vi "CSTK_MCListbox_Designer.vi"(10 "应用程序:菜单启动:VI":string, 11 "应用程序引用（本地）":refnum<vi>) -> ()   [LabVIEW 2015, in "CSTK_MCListbox Designer.lvlib"]
uses:
  CSTK_MCListbox Designer.lvlib
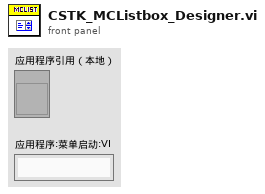
[diagram p1: front panel]
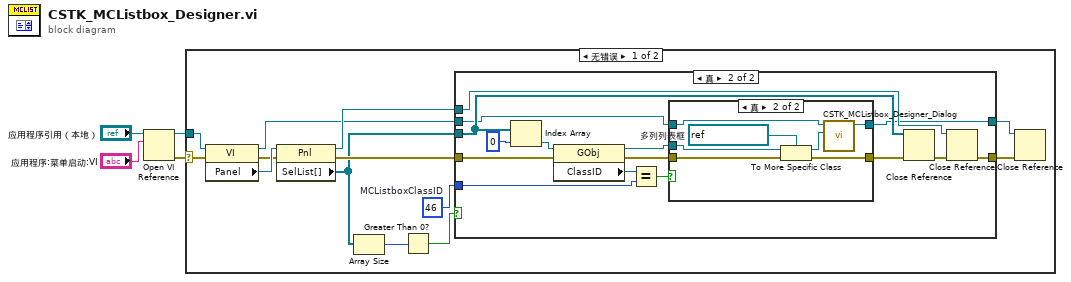
[diagram p0: block diagram]
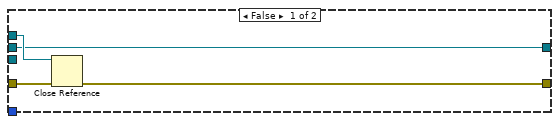
[diagram p2: hidden frame]
diagram:
  n1 = Open VI Reference(application reference (local)="应用程序引用（本地）", vi path="应用程序:菜单启动:VI") -> (vi reference=w1:refnum<vi>, error out=w2:errorcluster)  [unwired: 4 in]
  n2 = case shown="无错误" w2 {
    selector: w2 -> [w8 _]
    tunnel: w1 -> [w9 _]
    frame No Error {
      w10 = u32 46  # MCListboxClassID
      n3 = property class="VI"(reference=w9, error in=w8) -> (reference out=w6:refnum<vi>, error out=w16:errorcluster, "Panel"=w17:refnum<vi>)
      n4 = property class="Pnl"(reference=w17, error in=w16) -> (reference out=w12:refnum<vi>, error out=w13:errorcluster, "SelList[]"=w11:refnum<vi>[])
      n5 = Array Size(array=w11) -> (size(s)=w15:i32)
      n6 = Greater Than 0?(x=w15) -> (x > 0?=w14:bool)
      n7 = case shown="真" w14 {
        tunnel: w13 -> [w21 w34]
        tunnel: w12 -> [w20 w26]
        tunnel: w11 -> [_ w27]
        tunnel: w10 -> [_ w32]
        tunnel: [w19 w25] -> w7
        tunnel: w6 -> [w18 w23]
        tunnel: [w18 w22] -> w5
        frame False {
          n8 = Close Reference(reference=w20, error in (no error)=w21) -> (error out=w19:errorcluster)
        }
        frame True {
          n9 = Index Array(array=w27, index=0 ("索引")) -> (element=w35:refnum<vi>)
          n10 = property class="GObj"(reference=w35, error in=w34) -> (reference out=w24:refnum<vi>, error out=w30:errorcluster, "ClassID"=w33:u32)
          n11 = Equal?(x=w33, y=w32) -> (x = y?=w31:bool)
          n12 = case shown="真" w31 {
            tunnel: [w38 w41] -> w28
            tunnel: w30 -> [w38 w44]
            tunnel: w24 -> [_ w43]
            tunnel: w23 -> [w37 w40]
            tunnel: [w37 w39] -> w22
            frame False {
            }
            frame True {
              w45 = refnum<vi> refnum  # 多列列表框
              n13 = To More Specific Class(target class=w45, reference=w43, error in=w44) -> (specific class reference=w42:refnum<vi>, error out=w41:errorcluster)
              n14 = call "CSTK_MCListbox_Designer_Dialog.vi"("MCListbox引用句柄"=w42, "VI引用输入"=w40) -> ("VI引用输出"=w39:refnum<vi>)  [unwired: 9 in]
            }
          }
          n15 = Close Reference(reference=w27, error in (no error)=w28) -> (error out=w29:errorcluster)
          n16 = Close Reference(reference=w26, error in (no error)=w29) -> (error out=w25:errorcluster)
        }
      }
      n17 = Close Reference(reference=w5, error in (no error)=w7) -> ()  [unwired: 1 out]
    }
    frame Error {
    }
  }
